vi "Panel Get External_Q.vi"(8 "error in (no error)":errorcluster, 11 "Panel in":refnum<class "Panel Controller Interface.lvclass">) -> (0 "error out":errorcluster, 2 "External_Q":refnum<class "Message Enqueuer.lvclass">, 3 "Panel out":refnum<class "Panel Controller Interface.lvclass">)   [LabVIEW 2015, in "EditPanel API.lvlib" / "Panel Controller Interface.lvclass"]
uses:
  Panel Controller Interface.lvclass
  <vilib>/ActorFramework/Message Enqueuer/Message Enqueuer.lvclass
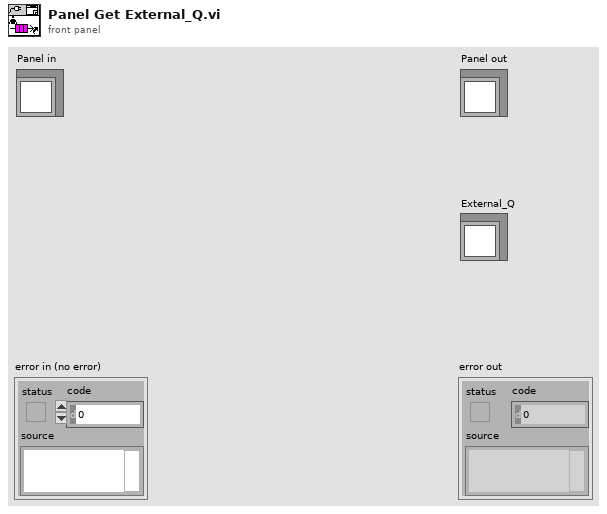
[diagram p1: front panel]
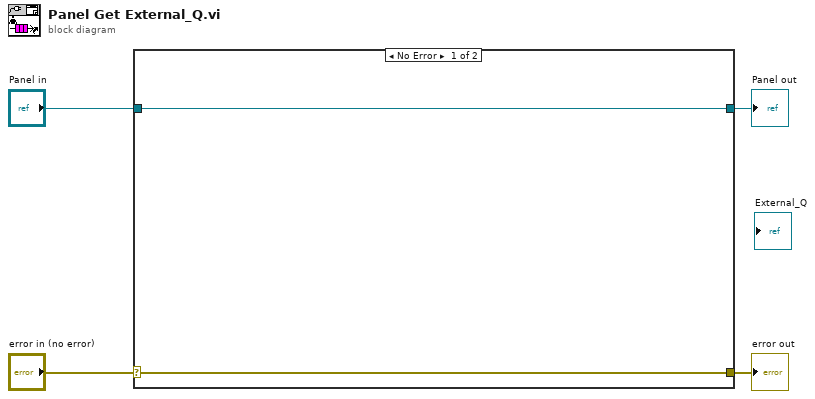
[diagram p0: block diagram]
diagram:
  n1 = case shown="No Error" "error in (no error)" {
    selector: "error in (no error)" -> [w5 w8]
    tunnel: [w5 w8] -> w3
    tunnel: [w6 w7] -> w1
    tunnel: "Panel in" -> [w6 w7]
    frame No Error {
    }
    frame Error {
    }
  }
  "error out" <- w3
  "Panel out" <- w1
